vi "Transaction ID Test.vi"() -> ()   [LabVIEW 2012]
uses:
  <vilib>/NI/Modbus Library/Data Model/Device Data Model.lvclass
  MB_ADU_TCP/MB_ADU_TCP.lvclass
  MB_Master_TCP/MB_Master_TCP.lvclass
  MB_ADU_TCP/MB_ADU_TCP.lvclass/MB_ADU_TCP.ctl
  <vilib>/NI/Modbus Library/API/Slave/Modbus Slave.lvclass
  MB_ADU_TCP/Read Transaction ID.vi
  <vilib>/NI/Modbus Library/API/Wrapper/Create TCP Slave.vi
  MB_ADU/MB_ADU.lvclass
  <vilib>/NI/Modbus Library/API/Wrapper/API Main.lvlib
  MB Master.lvlib
panel:
  out "Transaction ID 2":u16
  in  "stop 3":bool
  in  "stop 2":bool
  out "Transaction ID":u16
  in  "stop":bool
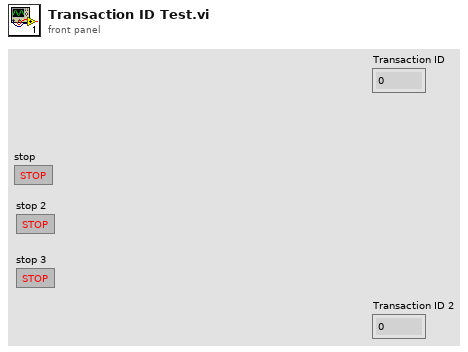
[diagram p1: front panel]
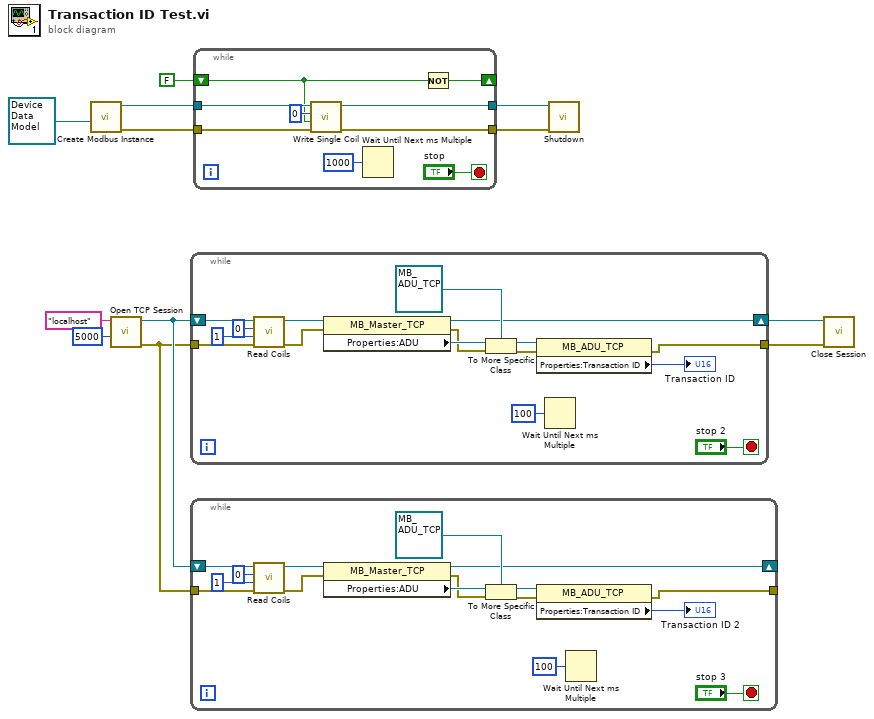
[diagram p0: block diagram]
diagram:
  n1 = call-poly <vilib>:"Create Modbus Instance.vi"("device data model"=refnum<class "Device Data Model.lvclass"> refnum) -> ("error out"=w10:errorcluster, "TCP slave instance"=w11:refnum<class "Modbus Slave.lvclass">)  [unwired: 9 in]
  n2 = call "Open TCP Session.vi"("Timeout (10000)"=5000, "IP Address"="localhost") -> ("error out"=w1:errorcluster, "MB_TCP session"=w2:refnum<class "MB_Master_TCP.lvclass">)  [unwired: 8 in]
  n3 = while {
    tunnel: w1 -> [w27]
    shift-right: [w16] -> w4
    shift-left: w2 -> [w28]
    tunnel: [w14] -> w3
    stop <- "stop 2" stop-if-true
    n4 = call "Read Coils.vi"("error in (no error)"=w27, "quantity"=u16 1, "starting address"=u16 0, "MB session in"=w28) -> ("error out"=w23:errorcluster, "MB session out"=w24:refnum<class "MB_Master_TCP.lvclass">)  [unwired: 5 in, 1 out]
    n5 = property class="MB_Master_TCP"(reference=w24, error in=w23) -> (reference out=w16:refnum<class "MB_Master_TCP.lvclass">, error out=w21:errorcluster, "Properties:ADU"=w22:refnum<class "MB_ADU.lvclass">)
    n6 = To More Specific Class(target class=refnum<class "MB_ADU_TCP.lvclass"> refnum ("MB Serial Master:MB_ADU_TCP"), reference=w22, error in=w21) -> (specific class reference=w19:refnum<class "MB_ADU_TCP.lvclass">, error out=w18:errorcluster)
    n7 = property class="MB_ADU_TCP"(reference=w19, error in=w18) -> (error out=w14:errorcluster, "Properties:Transaction ID"=→"Transaction ID":u16)  [unwired: 1 out]
    n8 = Wait Until Next ms Multiple(millisecond multiple=u32 100) -> ()  [unwired: 1 out]
  }
  n9 = while {
    tunnel: w1 -> [w43]
    shift-right: [w32] -> _
    shift-left: w2 -> [w44]
    tunnel: [w30] -> _
    stop <- "stop 3" stop-if-true
    n10 = call "Read Coils.vi"("error in (no error)"=w43, "quantity"=u16 1, "starting address"=u16 0, "MB session in"=w44) -> ("error out"=w39:errorcluster, "MB session out"=w40:refnum<class "MB_Master_TCP.lvclass">)  [unwired: 5 in, 1 out]
    n11 = property class="MB_Master_TCP"(reference=w40, error in=w39) -> (reference out=w32:refnum<class "MB_Master_TCP.lvclass">, error out=w37:errorcluster, "Properties:ADU"=w38:refnum<class "MB_ADU.lvclass">)
    n12 = To More Specific Class(target class=refnum<class "MB_ADU_TCP.lvclass"> refnum ("MB Serial Master:MB_ADU_TCP"), reference=w38, error in=w37) -> (specific class reference=w35:refnum<class "MB_ADU_TCP.lvclass">, error out=w34:errorcluster)
    n13 = property class="MB_ADU_TCP"(reference=w35, error in=w34) -> (error out=w30:errorcluster, "Properties:Transaction ID"=→"Transaction ID 2":u16)  [unwired: 1 out]
    n14 = Wait Until Next ms Multiple(millisecond multiple=u32 100) -> ()  [unwired: 1 out]
  }
  n15 = while {
    tunnel: w11 -> [w53]
    tunnel: w10 -> [w52]
    tunnel: [w50] -> w9
    tunnel: [w49] -> w8
    shift-right: [w47] -> _
    shift-left: FALSE -> [w46]
    stop <- "stop" stop-if-true
    n16 = call-dynamic "Write Single Coil.vi"("error in"=w52, "coil to write"=w46, "address"=u16 0, "Modbus slave in"=w53) -> ("error out"=w49:errorcluster, "Modbus slave out"=w50:refnum<class "Modbus Slave.lvclass">)  [unwired: 6 in]
    n17 = Wait Until Next ms Multiple(millisecond multiple=u32 1000) -> ()  [unwired: 1 out]
    n18 = Not(x=w46) -> (.not. x?=w47:bool)
  }
  n19 = call-dynamic "Shutdown.vi"("error in"=w8, "Modbus slave in"=w9) -> ()  [unwired: 9 in, 1 out]
  n20 = call-dynamic "Close Session.vi"("error in (no error)"=w3, "MB TCP session"=w4) -> ()  [unwired: 9 in, 1 out]
